vi "Prevent over 1024 lines.vi"(6 "Number of ROI":i32, 8 "New number of lines to be added (1)":i32=1, 9 "X-Y-Z coordinates":T1 {"ROI group ID" format="%#_6f"; "Laser Power (%)" format="%#_6f"; "Zoom" format="%#_6f"; "Frame Size" format="%#_6f"; "Number of lines" format="%#_6f"; "Composite ID" format="%#_6f"; "Angle (deg)" format="%#_6f"; "ROI Time (ns)" format="%#_6f"; "ROI ID" format="%#_6f"; "Pixels in ROI" format="%#_6f"; "ROI index" format="%#_6f"; "Z stop" format="%#_6f"; "Y stop" format="%#_6f"; "X stop" format="%#_6f"; "Z start" format="%#_6f"; "X start" format="%#_6f"; "Y start" format="%#_6f"}, 10 "Array in":T1[](array[typedef]) {"ROI group ID" format="%#_6f"; "Laser Power (%)" format="%#_6f"; "Zoom" format="%#_6f"; "Frame Size" format="%#_6f"; "Number of lines" format="%#_6f"; "Composite ID" format="%#_6f"; "Angle (deg)" format="%#_6f"; "ROI Time (ns)" format="%#_6f"; "ROI ID" format="%#_6f"; "Pixels in ROI" format="%#_6f"; "ROI index" format="%#_6f"; "Z stop" format="%#_6f"; "Y stop" format="%#_6f"; "X stop" format="%#_6f"; "Z start" format="%#_6f"; "X start" format="%#_6f"; "Y start" format="%#_6f"}, 11 "Existing number of lines across all ROI":i32) -> (1 "Exceeded 1024 lines":bool, 2 "Array out":T1[](array[typedef]) {"ROI group ID" format="%#_6f"; "Laser Power (%)" format="%#_6f"; "Zoom" format="%#_6f"; "Frame Size" format="%#_6f"; "Number of lines" format="%#_6f"; "Composite ID" format="%#_6f"; "Angle (deg)" format="%#_6f"; "ROI Time (ns)" format="%#_6f"; "ROI ID" format="%#_6f"; "Pixels in ROI" format="%#_6f"; "ROI index" format="%#_6f"; "Z stop" format="%#_6f"; "Y stop" format="%#_6f"; "X stop" format="%#_6f"; "Z start" format="%#_6f"; "X start" format="%#_6f"; "Y start" format="%#_6f"}, 3 "Resulting number of lines across all ROI":i32, 4 "Number of ROI":i32, 5 "Hardware limitation (number of lines across al ROI)":i32=1024)   [LabVIEW 2013]
uses:
  User Interface/Visualisation/Functional Imaging Viewer/Typedefs/ROI parameters data type.ctl
  Global Variables/General Globals.vi
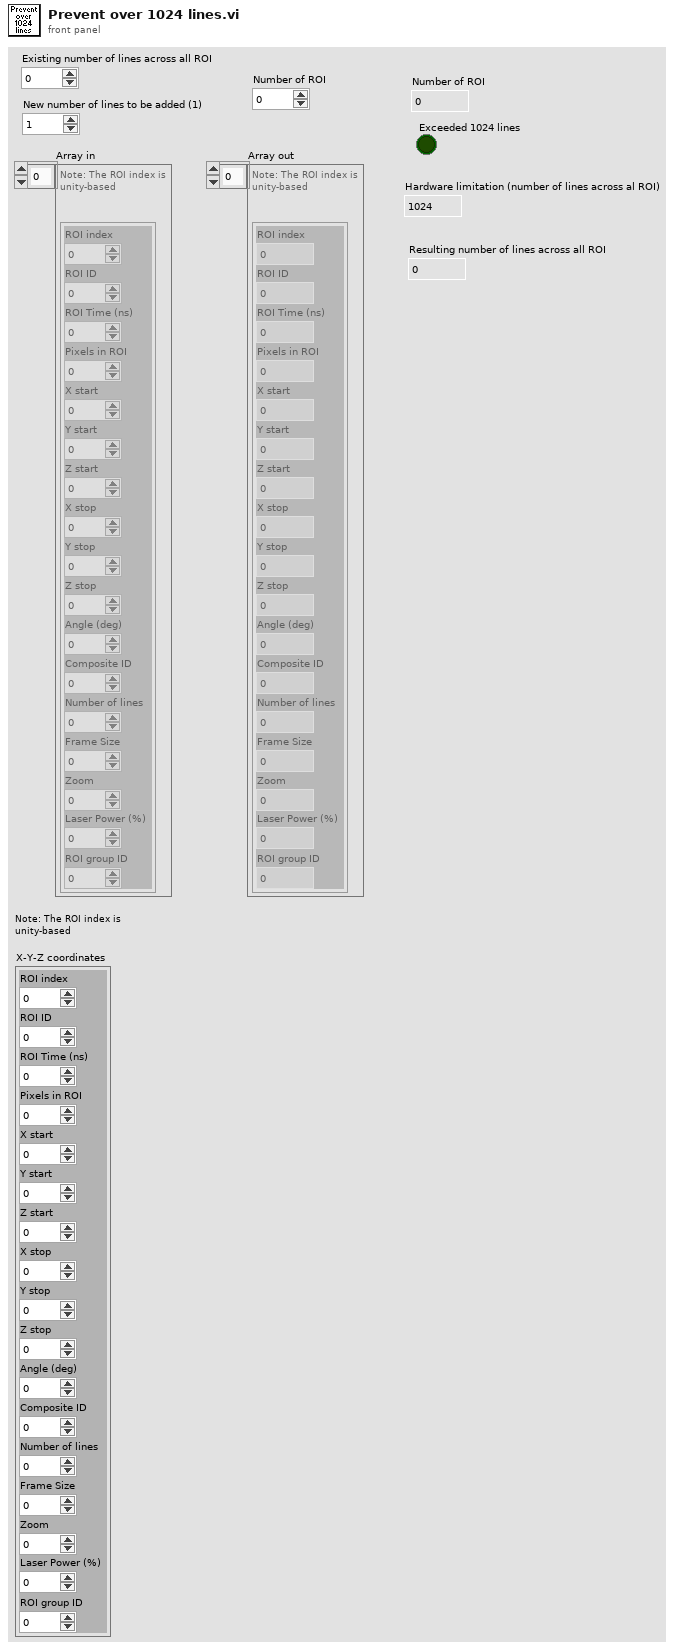
[diagram p1: front panel]
types:
  T1 = typedef "ROI parameters data type.ctl" = cluster{"ROI index":dbl, "ROI ID":dbl, "ROI Time (ns)":dbl, "Pixels in ROI":dbl, "X start":dbl, "Y start":dbl, "Z start":dbl, "X stop":dbl, "Y stop":dbl, "Z stop":dbl, "Angle (deg)":dbl, "Composite ID":dbl, "Number of lines":dbl, "Frame Size":dbl, "Zoom":dbl, "Laser Power (%)":dbl, "ROI group ID":dbl}
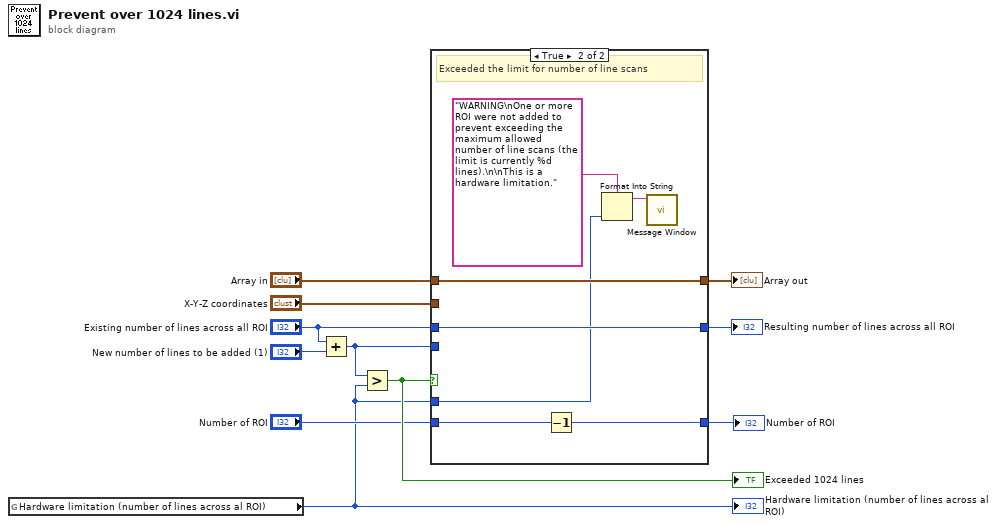
[diagram p0: block diagram]
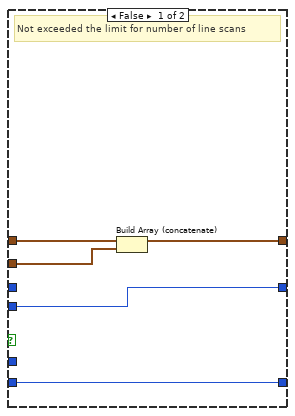
[diagram p2: hidden frame]
diagram:
  n1 = global read "General Globals.vi" "Hardware limitation (number of lines across al ROI)"() -> (w1:i32)
  "Hardware limitation (number of lines across al ROI)" <- w1
  n2 = Add(x="Existing number of lines across all ROI", y="New number of lines to be added (1)") -> (x+y=w4:i32)
  n3 = Greater?(x=w4, y=w1) -> (0:w10:bool)
  "Exceeded 1024 lines" <- w10
  n4 = case shown="True" w10 {
    tunnel: "Array in" -> [w16 w23]
    tunnel: [w15 w23] -> w8
    tunnel: "X-Y-Z coordinates" -> [w14 _]
    tunnel: "Existing number of lines across all ROI" -> [_ w22]
    tunnel: [w13 w22] -> w5
    tunnel: w4 -> [w13 _]
    tunnel: "Number of ROI" -> [w12 w21]
    tunnel: [w12 w20] -> w2
    tunnel: w1 -> [_ w17]
    frame False {
      # "Not exceeded the limit for number of line scans"
      n5 = Build Array (concatenate)(w16, w14) -> (w15:T1[])
    }
    frame True {
      # "Exceeded the limit for number of line scans"
      n6 = Decrement(x=w21) -> (x-1=w20:i32)
      n7 = Format Into String(format string="WARNING\nOne or more ROI were not added to prevent exceeding the maximum allowed number of line scans (the limit is currently %d lines).\n\nThis is a hardware limitation." ("message"), w17) -> (resulting string=w18:string)  [unwired: 2 in, 1 out]
      n8 = call "Message Window.vi"("Message string"=w18) -> ()  [unwired: 10 in, 1 out]
    }
  }
  "Array out" <- w8
  "Resulting number of lines across all ROI" <- w5
  "Number of ROI" <- w2
